vi "new DoorNeedingSpell.vi"(8 "error in (no error)":errorcluster, 9 "r2":refnum<data-value>, 10 "r1":refnum<data-value>) -> (0 "error out":errorcluster, 3 "DoorNeedingSpell* out":T1)   [LabVIEW 2016, in "DoorNeedingSpell.lvclass"]
uses:
  DoorNeedingSpell.lvclass
  Base/Room/Room.lvclass
  DoorNeedingSpell Reference.ctl
  C:/github/LVOOP-creational-patterns/Maze-Classes/src/Base/Door/Door.lvclass
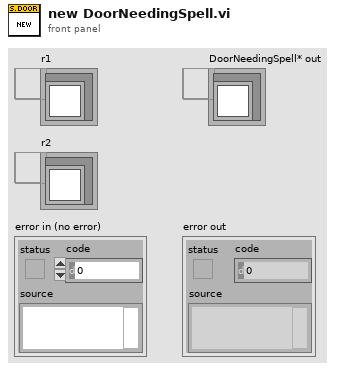
[diagram p1: front panel]
types:
  T1 = typedef "DoorNeedingSpell.lvclass/DoorNeedingSpell Reference.ctl" = refnum<data-value>
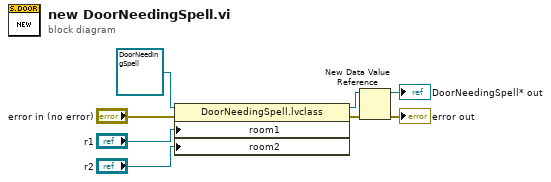
[diagram p0: block diagram]
diagram:
  n1 = property class="DoorNeedingSpell.lvclass"(reference=refnum<class "DoorNeedingSpell.lvclass"> refnum ("DoorNeedingSpell in"), error in="error in (no error)", "room1"="r1", "room2"="r2") -> (reference out=w5:refnum<class "DoorNeedingSpell.lvclass">, error out=w4:errorcluster)
  n2 = New Data Value Reference(data value=w5, error in=w4) -> (data value reference=→"DoorNeedingSpell* out":refnum<data-value>, error out=→"error out":errorcluster)
